vi "Simple Client - Init.vi"(0 "Process Variable":string caption="Process Variable to Read (Numeric Only)", 5 "Host":string="localhost" caption="IOC Host", 7 "Process Name for\nthis particular VI":string) -> (15 "error out":errorcluster)   [LabVIEW 2011]
uses:
  <vilib>/variable/tagger/epics/API/NI_EPICS_Client.lvlib
  <vilib>/lvdsc/NI_DSC.lvlib
  Program Files (x86)/National Instruments/LabVIEW 2011/resource/objmgr/nvio.rc
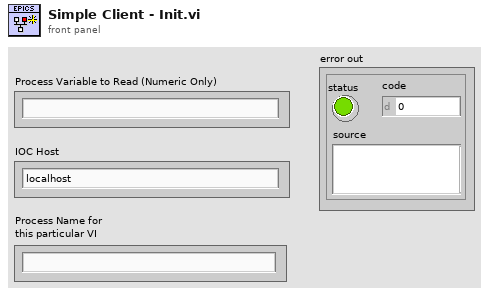
[diagram p1: front panel]
types:
  T1 = enum32{"u32BitField", "bool", "double", "string", "int8", "uint8", "int16", "uint16", "int32", "uint32", "int64", "uint64", "single", "double waveform", "int16 waveform", "array of boolean", "array of int8", "array of uint8", "array of int16", "array of uint16", "array of int32", "array of uint32", "array of int64", "array of uint64", "array of single", "array of double", "array of double waveform", "array of int16 waveform", "array of string", "variant", "timestamp", "fixed point", "custom"}
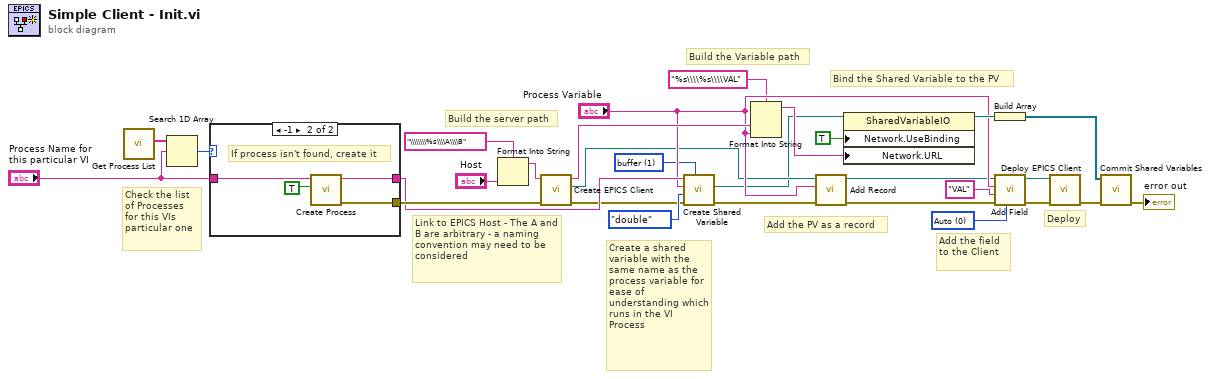
[diagram p0: block diagram]
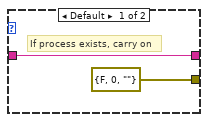
[diagram p2: hidden frame]
diagram:
  w1 = u16 1 items=["commit", "buffer"] ("set mode")
  w11 = u16 0 items=["Auto", "Double", "Bool", "String", "Short", "Float", "Enum", "Long", "Array of Double"] ("data type")
  # "Deploy"
  # "Add the field to the Client"
  # "Bind the Shared Variable to the PV"
  # "Add the PV as a record"
  # "Build the Variable path"
  # "Build the server path"
  # "Create a shared variable with the same name as the process variable for ease of understanding which runs in the VI Process"
  # "Link to EPICS Host - The A and B are arbitrary - a naming convention may need to be considered"
  # "Check the list of Processes for this VIs particular one"
  n1 = call <vilib>:"Get Process List.vi"() -> ("processes"=w22:string[])  [unwired: 10 in, 1 out]
  n2 = Search 1D Array(1D array=w22, element="Process Name for\nthis particular VI") -> (index of element=w23:i32)  [unwired: 1 in]
  n3 = case shown="-1" w23 {
    tunnel: [w31 w34] -> w24
    tunnel: [errorcluster {"status"=FALSE, "code"=0, "source"=""} ("error out") w33] -> w25
    tunnel: "Process Name for\nthis particular VI" -> [w31 w32]
    frame Default {
      # "If process exists, carry on"
    }
    frame -1 {
      # "If process isn't found, create it"
      n4 = call <vilib>:"Create Process.vi"("run?"=TRUE, "process name"=w32) -> ("error out"=w33:errorcluster, "process name out"=w34:string)  [unwired: 8 in]
    }
  }
  n5 = Format Into String(format string="\\\\\\\\%s\\\\A\\\\B" ("EPICS Client URL in"), "Host") -> (resulting string=w14:string)  [unwired: 2 in, 1 out]
  n6 = call <vilib>:"Create EPICS Client.vi"("error in (no error)"=w25, "EPICS Client URL in"=w14) -> ("error out"=w9:errorcluster, "EPICS Client ref"=w8:refnum<data-value>, "EPICS Client URL out"=w27:string)  [unwired: 7 in]
  n7 = call <vilib>:"Create Shared Variable.vi"("set mode"=w1, "error in (no error)"=w9, "data type"=T1."double", "shared variable name"="Process Variable", "process name"=w24) -> ("error out"=w6:errorcluster, "shared variable"=w4:refnum<k21>)  [unwired: 4 in, 1 out]
  n8 = Format Into String(format string="%s\\\\%s\\\\VAL" ("EPICS Client URL in"), w27, "Process Variable") -> (resulting string=w19:string)  [unwired: 2 in, 1 out]
  n9 = call <vilib>:"Add Record.vi"("error in (no error)"=w6, "record name"="Process Variable", "EPICS Client ref in"=w8) -> ("error out"=w5:errorcluster, "EPICS Client ref out"=w7:refnum<data-value>)  [unwired: 5 in, 2 out]
  n10 = property class="SharedVariableIO"(reference=w4, "Network.UseBinding"=TRUE ("use binding? (F)"), "Network.URL"=w19) -> (reference out=w21:refnum<k21>)  [unwired: 1 in, 1 out]
  n11 = Build Array(w21) -> (w2:refnum<k21>[])
  n12 = call <vilib>:"Add Field.vi"("data type"=w11, "error in (no error)"=w5, "field name"="VAL", "record name"="Process Variable", "EPICS Client ref in"=w7) -> ("error out"=w29:errorcluster, "EPICS Client ref out"=w28:refnum<data-value>)  [unwired: 3 in, 2 out]
  n13 = call <vilib>:"Deploy EPICS Client.vi"("error in (no error)"=w29, "EPICS Client ref in"=w28) -> ("error out"=w20:errorcluster)  [unwired: 8 in, 1 out]
  n14 = call <vilib>:"Commit Shared Variables.vi"("error in (no error)"=w20, "shared variables"=w2) -> ("error out"=→"error out":errorcluster)  [unwired: 8 in, 1 out]
